vi "LiquidFlowOut.vi"(10 "level_decrease_in_points":i32, 11 "liquid_temperature":dbl[][](array[numeric])) -> (3 "new_liquid_temperature":dbl[][](array[numeric]))   [LabVIEW 2020]
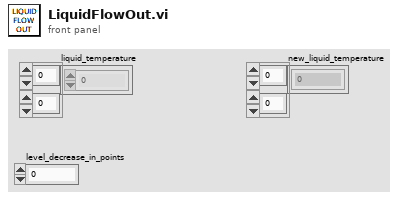
[diagram p1: front panel]
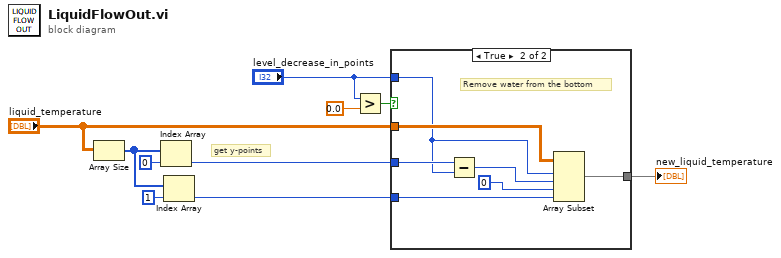
[diagram p0: block diagram]
diagram:
  # "get y-points"
  n1 = Array Size(array="liquid_temperature") -> (size(s)=w7:i32[])
  n2 = Index Array(array=w7, index=0) -> (element=w9:i32)
  n3 = Index Array(array=w7, index=1) -> (element=w6:i32)
  n4 = Greater?(x="level_decrease_in_points", y=0.0) -> (0:w5:bool)
  n5 = case shown="True" w5 {
    tunnel: "liquid_temperature" -> [w11 w17]
    tunnel: [w11 w12] -> w2
    tunnel: w9 -> [_ w15]
    tunnel: w6 -> [_ w13]
    tunnel: "level_decrease_in_points" -> [_ w14]
    frame False {
    }
    frame True {
      # "Remove water from the bottom"
      n6 = Subtract(x=w15, y=w14) -> (x-y=w16:i32)
      n7 = Array Subset(array=w17, index (row)=w14, length (row)=w16, index (col)=0 ("index"), length (col)=w13) -> (w12:dbl[][])
    }
  }
  "new_liquid_temperature" <- w2
